vi "preprocess.vi"(8 "error in (no error)":errorcluster, 10 "image file path":path, 11 "GenericSegmenter in":refnum<class "GenericSegmenter.lvclass">) -> (0 "error out":errorcluster, 2 "preprocessed file path":path, 3 "GenericSegmenter out":refnum<class "GenericSegmenter.lvclass">)   [LabVIEW 2010, in "GenericSegmenter.lvclass"]
uses:
  GenericSegmenter.lvclass
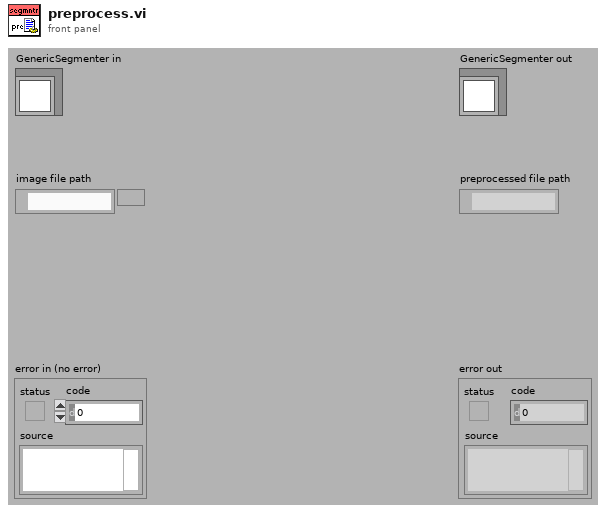
[diagram p1: front panel]
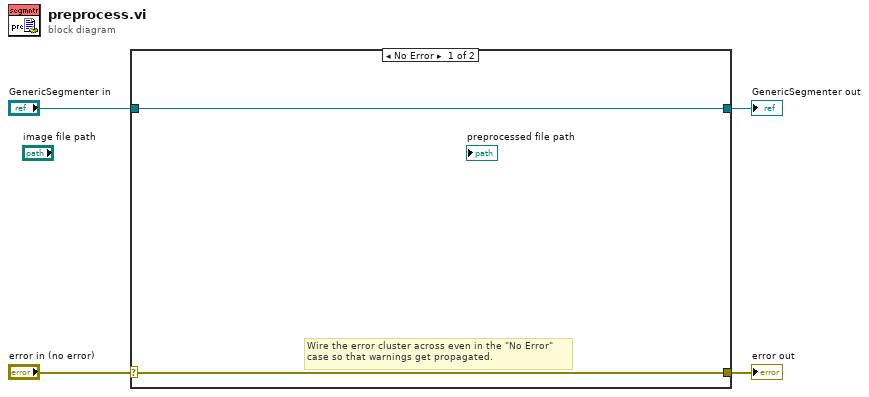
[diagram p0: block diagram]
diagram:
  n1 = case shown="No Error" "error in (no error)" {
    selector: "error in (no error)" -> [w5 w8]
    tunnel: [w5 w8] -> w3
    tunnel: [w6 w7] -> w1
    tunnel: "GenericSegmenter in" -> [w6 w7]
    frame No Error {
      # "Wire the error cluster across even in the \"No Error\"\ncase so that warnings get propagated."
    }
    frame Error {
    }
  }
  "error out" <- w3
  "GenericSegmenter out" <- w1
